vi "FindRowIndex.vi"(8 "error in (no error)":errorcluster, 9 "PartNumberData":T1(array[cluster]), 10 "Barcode":string) -> (0 "error out":errorcluster, 1 "SerialNumber":string, 2 "PartNumber":string, 3 "ArrayIndex":i32, 5 "ModelNumber":string)   [LabVIEW 2021]
uses:
  <vilib>/regexp/Match Regular Expression.xnode
panel:
  out "PN_SN":string
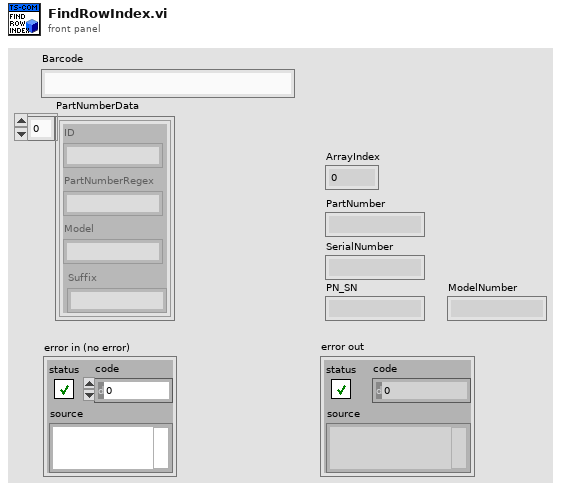
[diagram p1: front panel]
types:
  T1 = cluster{"ID":string, "PartNumberRegex":string, "Model":string, "Suffix":string}[]
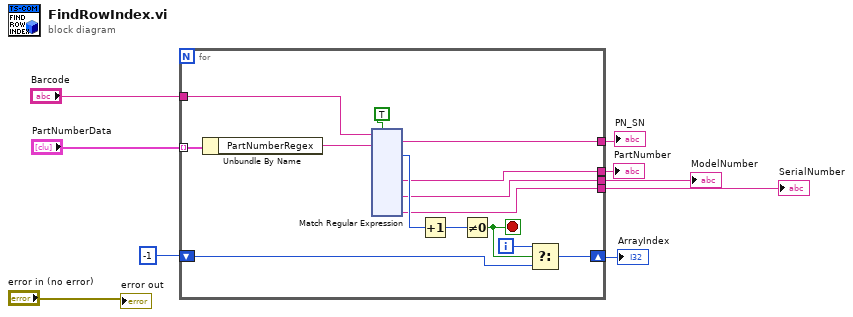
[diagram p0: block diagram]
diagram:
  n1 = for {
    tunnel: "Barcode" -> [w20]
    shift-right: [w16] -> w7
    shift-left: -1 -> [w17]
    tunnel: "PartNumberData" -> [w15] mode=indexing
    tunnel: [w12] -> w4
    tunnel: [w10] -> w3
    tunnel: [w13] -> w2
    tunnel: [w11] -> w1
    i -> [w18]
    stop <- w19 stop-if-true
    n2 = Unbundle By Name(w15) -> ("PartNumberRegex"=w14:string)
    n3 = xnode "Match Regular Expression"("input string"=w20, "regular expression"=w14, "ignore case? (F)"=TRUE) -> ("whole match"=w13:string, "offset past match"=w23:i32, "submatch 2"=w12:string, "submatch 4"=w11:string, "submatch 6"=w10:string)  [unwired: 3 in, 6 out]
    n4 = Increment(x=w23) -> (x+1=w22:i32)
    n5 = Not Equal To 0?(x=w22) -> (x != 0?=w19:bool)
    n6 = Select(t=w18, s=w19, f=w17) -> (s? t:f=w16:i32)
  }
  "ArrayIndex" <- w7
  "PartNumber" <- w4
  "SerialNumber" <- w3
  "PN_SN" <- w2
  "ModelNumber" <- w1
  "error out" <- "error in (no error)"
